vi "nelder_make_next_simplex.vi"(8 "error in":errorcluster, 9 "settling time":u32, 10 "input \nsimplex":T3={"Reflected"=[[13.898129, 13.898129, 12.898129], [13.103427, 14.103427, 13.103427]], "Expanded"=[[13.898129, 13.898129, 11.898129], [13.103427, 14.103427, 12.603427]], "Contracted inside"=[[13.898129, 13.898129, 13.398129], [13.103427, 14.103427, 13.353427]], "Contracted outside"=[[13.898129, 13.898129, 14.398129], [13.103427, 14.103427, 13.853427]], "Shrunk"=[[13.898129, 13.898129, 14.398129], [13.103427, 13.603427, 13.603427]]}, 11 "refs":T2) -> (0 "error out":errorcluster, 3 "next simplex":sgl[][](array[numeric]))   [LabVIEW 2018]
uses:
  C:/Program Files/National Instruments/LabVIEW 2018/instr.lib/IDS/ueye.NET/uEyeDotNet.dll
  <userlib>/PDamp/PDref.ctl
panel:
  out "worst":sgl
  out "second worst":sgl
  out "best":sgl
  out "reflected":dbl
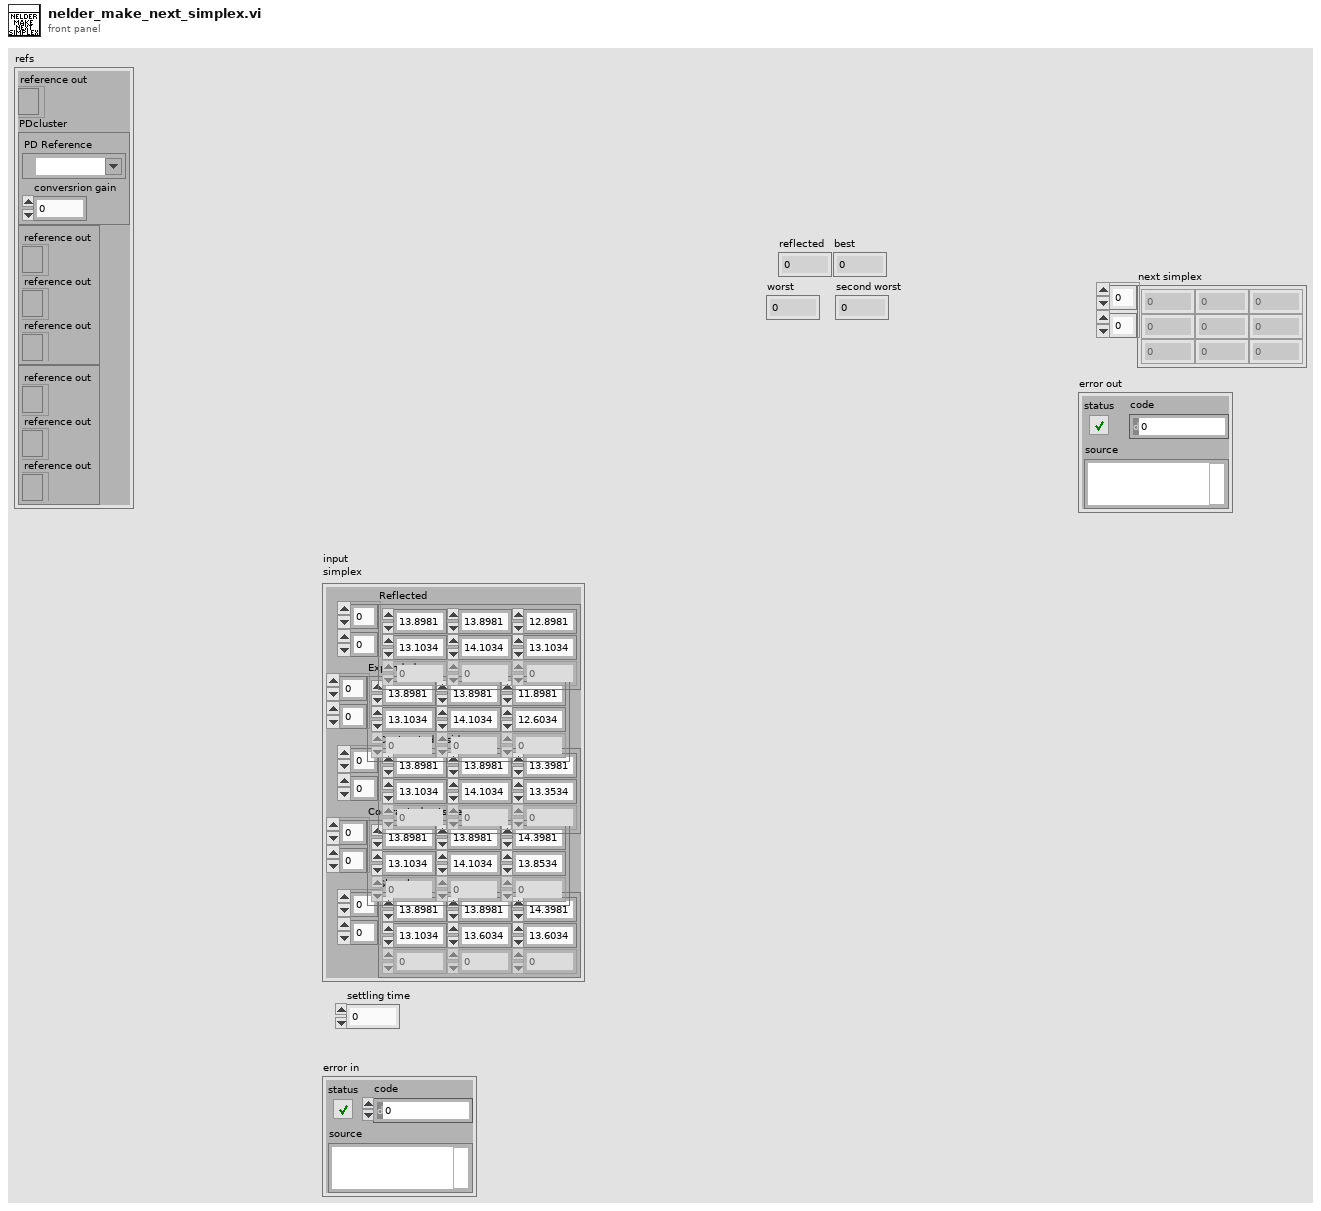
[diagram p1: front panel]
types:
  T1 = typedef "PDref.ctl" = cluster{"PD Reference":refnum<visa-resource-name>, "conversrion gain":dbl}
  T2 = cluster{"reference out":refnum<k24>, "PDcluster":T1, cluster{"reference out":refnum<k7>, "reference out":refnum<k7>, "reference out":refnum<k7>}, cluster{"reference out":refnum<k7>, "reference out":refnum<k7>, "reference out":refnum<k7>}}
  T3 = cluster{"Reflected":sgl[][], "Expanded":sgl[][], "Contracted inside":sgl[][], "Contracted outside":sgl[][], "Shrunk":sgl[][]}
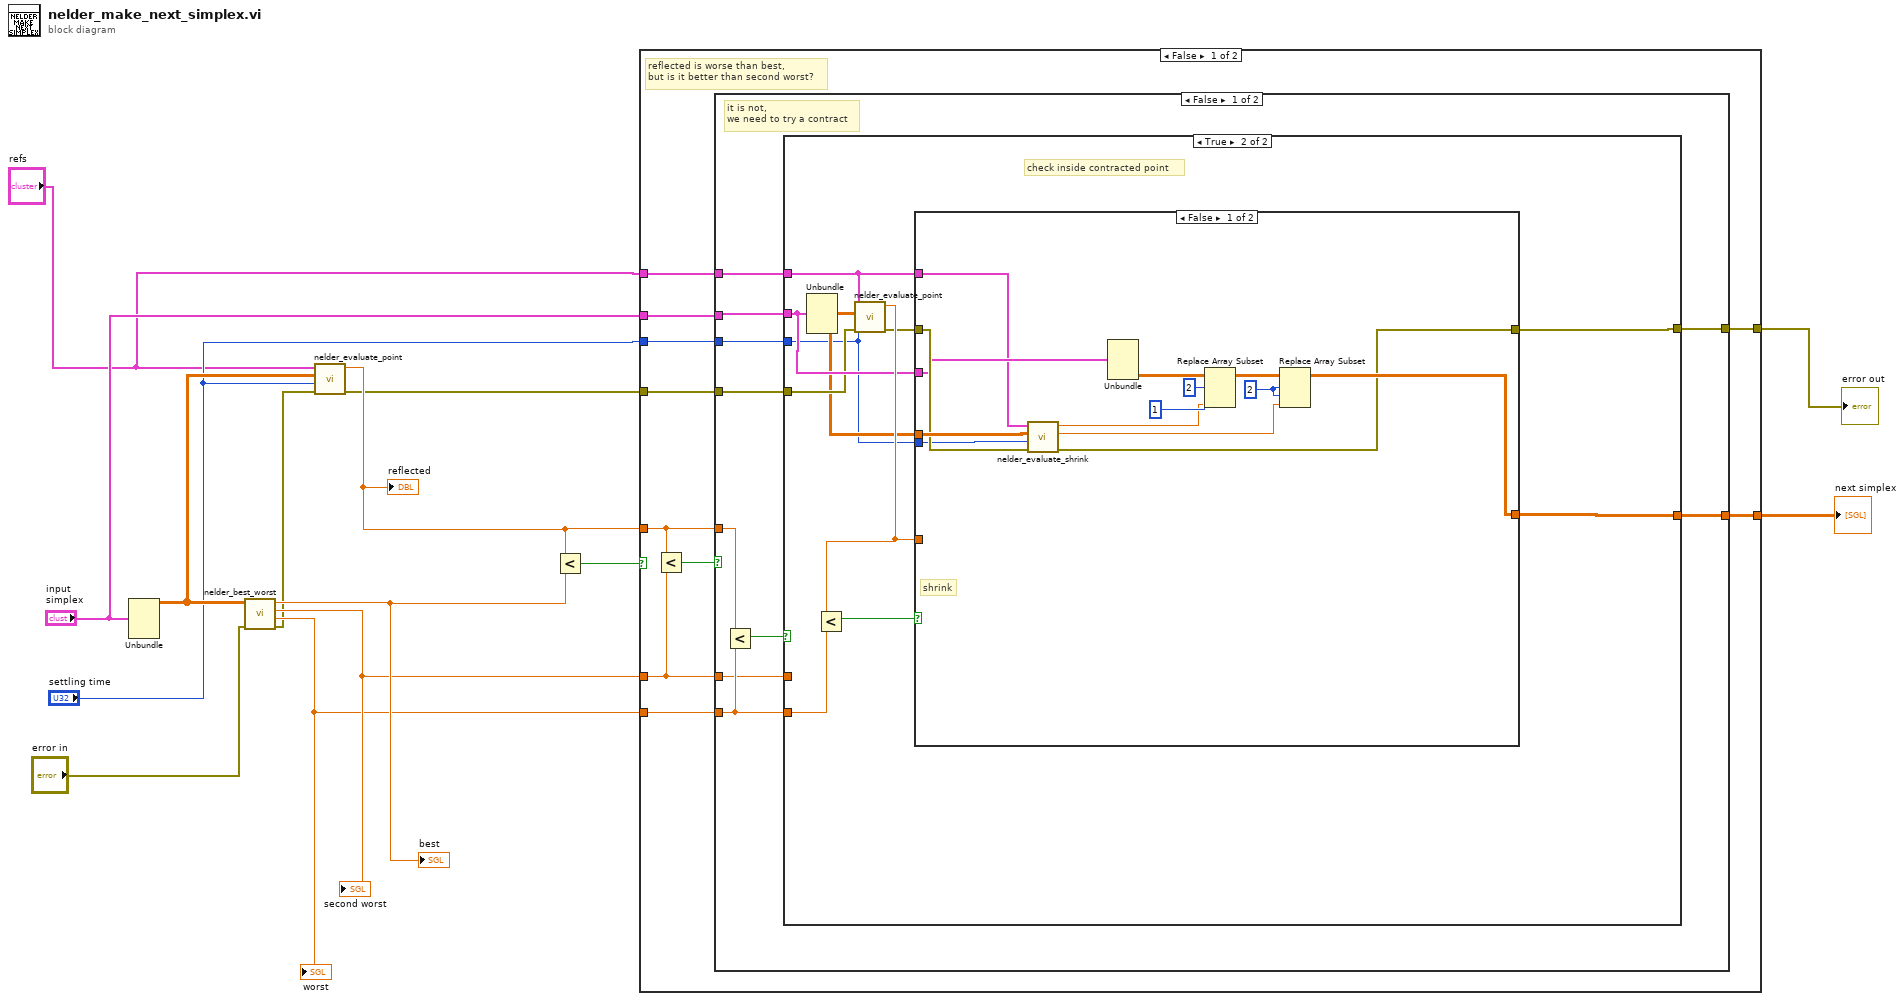
[diagram p0: block diagram]
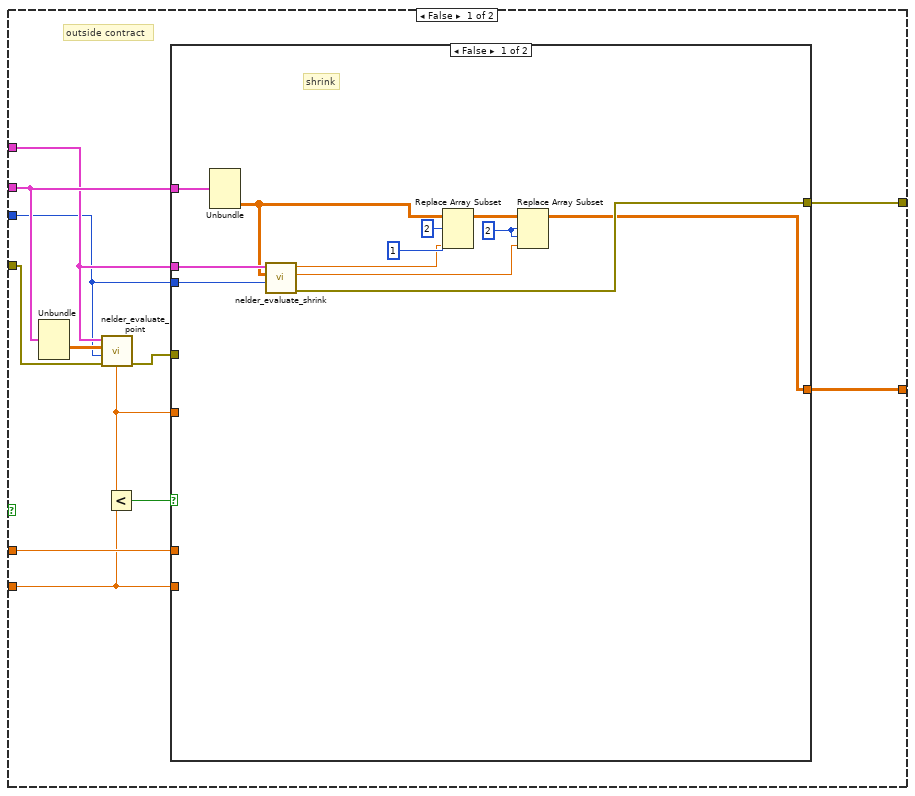
[diagram p2: hidden frame]
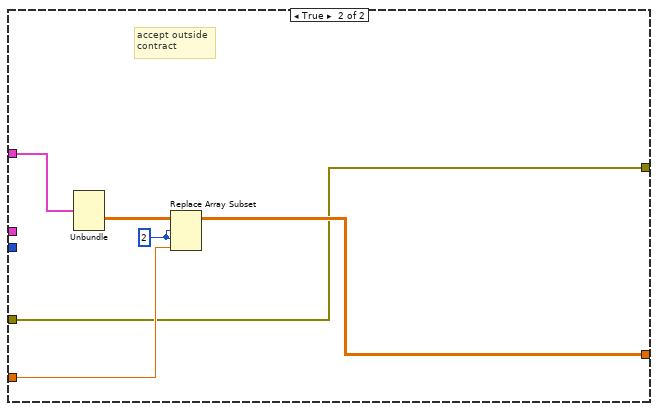
[diagram p3: hidden frame]
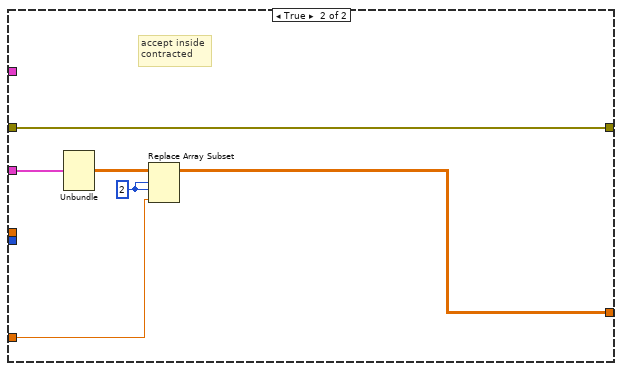
[diagram p4: hidden frame]
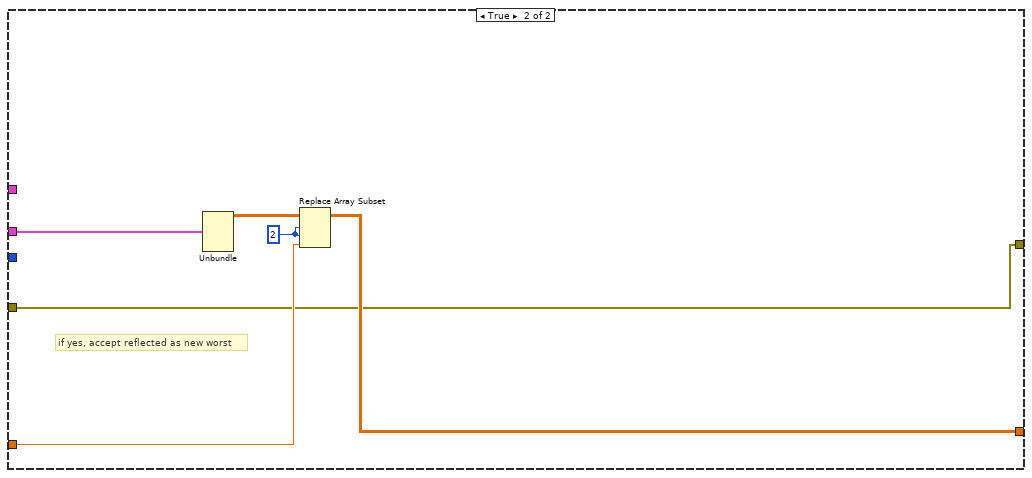
[diagram p5: hidden frame]
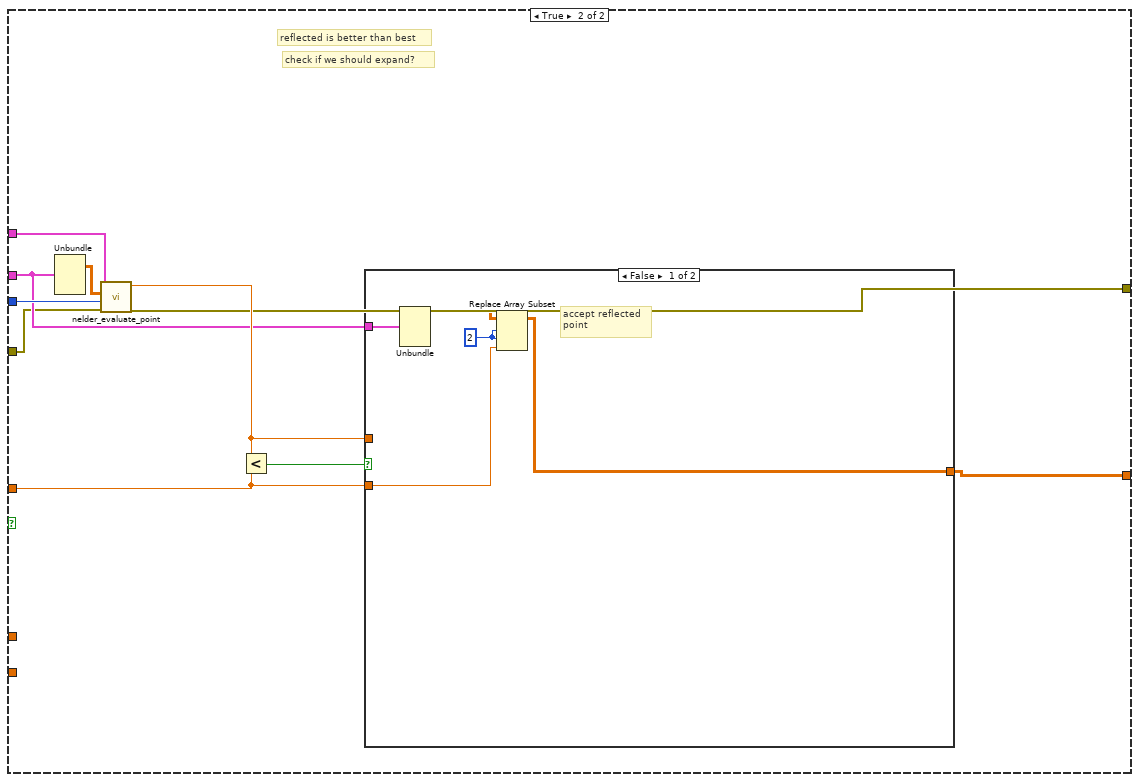
[diagram p6: hidden frame]
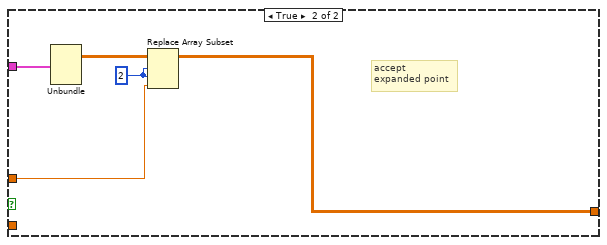
[diagram p7: hidden frame]
diagram:
  n1 = Unbundle("input \nsimplex") -> ("Reflected"=w13:sgl[][])  [unwired: 4 out]
  n2 = call "nelder_best_worst.vi"("error in"="error in", "array"=w13) -> ("error out"=w8:errorcluster, "worst"=w9:sgl, "second worst"=w10:sgl, "best"=w11:sgl)  [unwired: 6 in]
  "best" <- w11
  "second worst" <- w10
  "worst" <- w9
  n3 = call "nelder_evaluate_point.vi"("error in"=w8, "settling time"="settling time", "point"=w13, "refs"="refs") -> ("error out"=w3:errorcluster, "f_Val"=w12:dbl)  [unwired: 6 in]
  "reflected" <- w12
  n4 = Less?(x=w12, y=w11) -> (x < y?=w14:bool)
  n5 = case shown="False" w14 {
    tunnel: w12 -> [w23 w112]
    tunnel: w10 -> [w15 _]
    tunnel: w9 -> [w22 _]
    tunnel: [w21 w105] -> w6
    tunnel: "refs" -> [w19 w107]
    tunnel: "input \nsimplex" -> [w20 w106]
    tunnel: "settling time" -> [w18 w110]
    tunnel: w3 -> [w17 w104]
    tunnel: [w16 w103] -> w2
    frame False {
      # "reflected is worse than best,\nbut is it better than second worst?"
      n6 = Less?(x=w23, y=w15) -> (x < y?=w24:bool)
      n7 = case shown="False" w24 {
        tunnel: w23 -> [w34 w100]
        tunnel: w22 -> [w32 _]
        tunnel: [w28 w99] -> w21
        tunnel: w20 -> [w31 w98]
        tunnel: w19 -> [w30 _]
        tunnel: w18 -> [w29 _]
        tunnel: w17 -> [w27 w97]
        tunnel: [w26 w97] -> w16
        tunnel: w15 -> [w25 _]
        frame False {
          # "it is not, \nwe need to try a contract"
          n8 = Less?(x=w34, y=w32) -> (x < y?=w33:bool)
          n9 = case shown="True" w33 {
            tunnel: w32 -> [w39 w76]
            tunnel: [w37 w74] -> w28
            tunnel: w31 -> [w38 w71]
            tunnel: w30 -> [w36 w66]
            tunnel: w29 -> [w35 w65]
            tunnel: w27 -> [w44 w70]
            tunnel: [w42 w69] -> w26
            tunnel: w25 -> [w40 _]
            frame False {
              # "outside contract"
              n10 = Unbundle(w38) -> ("Contracted outside"=w45:sgl[][])  [unwired: 4 out]
              n11 = call "nelder_evaluate_point.vi"("error in"=w44, "settling time"=w35, "point"=w45, "refs"=w36) -> ("error out"=w43:errorcluster, "f_Val"=w41:dbl)  [unwired: 6 in]
              n12 = Less?(x=w41, y=w39) -> (x < y?=w46:bool)
              n13 = case shown="False" w46 {
                tunnel: w41 -> [_ w61]
                tunnel: w43 -> [_ w59]
                tunnel: [w49 w59] -> w42
                tunnel: w40 -> [_ _]
                tunnel: w39 -> [_ _]
                tunnel: w38 -> [w52 w63]
                tunnel: [w47 w60] -> w37
                tunnel: w36 -> [w51 _]
                tunnel: w35 -> [w50 _]
                frame False {
                  w54 = 2 ("index (col)")
                  # "shrink"
                  n14 = Unbundle(w52) -> ("Shrunk"=w48:sgl[][])  [unwired: 4 out]
                  n15 = call "nelder_evaluate_shrink.vi"("settling time"=w50, "shrink point"=w48, "Cluster"=w51) -> ("error out"=w49:errorcluster, "f_val2"=w53:dbl, "f_val1"=w56:dbl)  [unwired: 6 in]
                  n16 = Replace Array Subset(array=w48, new element=w56, index (row)=2 ("disabled index (row)"), index (col)=1 ("index (row)")) -> (w55:sgl[][])
                  n17 = Replace Array Subset(array=w55, new element=w53, index (row)=w54, index (col)=w54) -> (w47:sgl[][])
                }
                frame True {
                  w64 = 2 ("index (row)")
                  # "accept outside\ncontract"
                  n18 = Unbundle(w63) -> ("Contracted outside"=w62:sgl[][])  [unwired: 4 out]
                  n19 = Replace Array Subset(array=w62, new element=w61, index (row)=w64, index (col)=w64) -> (w60:sgl[][])
                }
              }
            }
            frame True {
              # "check inside contracted point"
              n20 = Unbundle(w71) -> ("Contracted inside"=w73:sgl[][], "Shrunk"=w67:sgl[][])  [unwired: 3 out]
              n21 = call "nelder_evaluate_point.vi"("error in"=w70, "settling time"=w65, "point"=w73, "refs"=w66) -> ("error out"=w68:errorcluster, "f_Val"=w72:dbl)  [unwired: 6 in]
              n22 = Less?(x=w72, y=w76) -> (x < y?=w75:bool)
              n23 = case shown="False" w75 {
                tunnel: [w80 w93] -> w74
                tunnel: w72 -> [_ w92]
                tunnel: w71 -> [w87 w95]
                tunnel: [w78 w91] -> w69
                tunnel: w68 -> [w89 w91]
                tunnel: w67 -> [w90 _]
                tunnel: w66 -> [w77 _]
                tunnel: w65 -> [w88 _]
                frame False {
                  w81 = 2 ("index (col)")
                  # "shrink"
                  n24 = call "nelder_evaluate_shrink.vi"("error in"=w89, "settling time"=w88, "shrink point"=w90, "Cluster"=w77) -> ("error out"=w78:errorcluster, "f_val2"=w79:dbl, "f_val1"=w83:dbl)  [unwired: 5 in]
                  n25 = Unbundle(w87) -> ("Shrunk"=w86:sgl[][])  [unwired: 4 out]
                  n26 = Replace Array Subset(array=w86, new element=w83, index (row)=2 ("disabled index (row)"), index (col)=1 ("index (row)")) -> (w82:sgl[][])
                  n27 = Replace Array Subset(array=w82, new element=w79, index (row)=w81, index (col)=w81) -> (w80:sgl[][])
                }
                frame True {
                  w96 = 2 ("index (row)")
                  # "accept inside\ncontracted"
                  n28 = Unbundle(w95) -> ("Contracted inside"=w94:sgl[][])  [unwired: 4 out]
                  n29 = Replace Array Subset(array=w94, new element=w92, index (row)=w96, index (col)=w96) -> (w93:sgl[][])
                }
              }
            }
          }
        }
        frame True {
          w101 = 2 ("index (row)")
          # "if yes, accept reflected as new worst"
          n30 = Unbundle(w98) -> ("Reflected"=w102:sgl[][])  [unwired: 4 out]
          n31 = Replace Array Subset(array=w102, new element=w100, index (row)=w101, index (col)=w101) -> (w99:sgl[][])
        }
      }
    }
    frame True {
      # "check if we should expand?"
      # "reflected is better than best"
      n32 = Unbundle(w106) -> ("Expanded"=w111:sgl[][])  [unwired: 4 out]
      n33 = call "nelder_evaluate_point.vi"("error in"=w104, "settling time"=w110, "point"=w111, "refs"=w107) -> ("error out"=w103:errorcluster, "f_Val"=w108:dbl)  [unwired: 6 in]
      n34 = Less?(x=w108, y=w112) -> (x < y?=w109:bool)
      n35 = case shown="False" w109 {
        tunnel: w108 -> [_ w119]
        tunnel: [w114 w118] -> w105
        tunnel: w112 -> [w113 _]
        tunnel: w106 -> [w116 w121]
        frame False {
          w117 = 2 ("index (row)")
          # "accept reflected \npoint"
          n36 = Unbundle(w116) -> ("Reflected"=w115:sgl[][])  [unwired: 4 out]
          n37 = Replace Array Subset(array=w115, new element=w113, index (row)=w117, index (col)=w117) -> (w114:sgl[][])
        }
        frame True {
          w122 = 2 ("index (row)")
          # "accept \nexpanded point"
          n38 = Unbundle(w121) -> ("Expanded"=w120:sgl[][])  [unwired: 4 out]
          n39 = Replace Array Subset(array=w120, new element=w119, index (row)=w122, index (col)=w122) -> (w118:sgl[][])
        }
      }
    }
  }
  "next simplex" <- w6
  "error out" <- w2
